vi "Round to 0.0001 (SubVI).vi"(11 "Input":dbl) -> (3 "Rounded output":dbl)   [LabVIEW 2018]
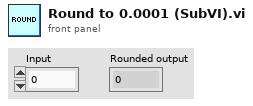
[diagram p1: front panel]
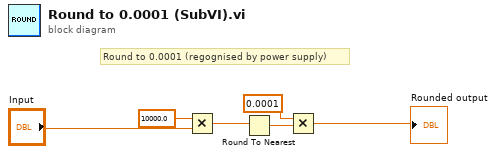
[diagram p0: block diagram]
diagram:
  # "Round to 0.0001 (regognised by power supply)"
  n1 = Multiply(x=10000.0, y="Input") -> (x*y=w2:dbl)
  n2 = Round To Nearest(number=w2) -> (nearest integer value=w3:dbl)
  n3 = Multiply(x=0.0001, y=w3) -> (x*y=→"Rounded output":dbl)
